vi "LEDShow.vi"(1 "DigntNumber":u32, 2 "InputNumber":dbl) -> (0 "MyLED":u16[](array[ring]))   [LabVIEW 2011]
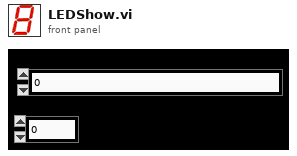
[diagram p1: front panel]
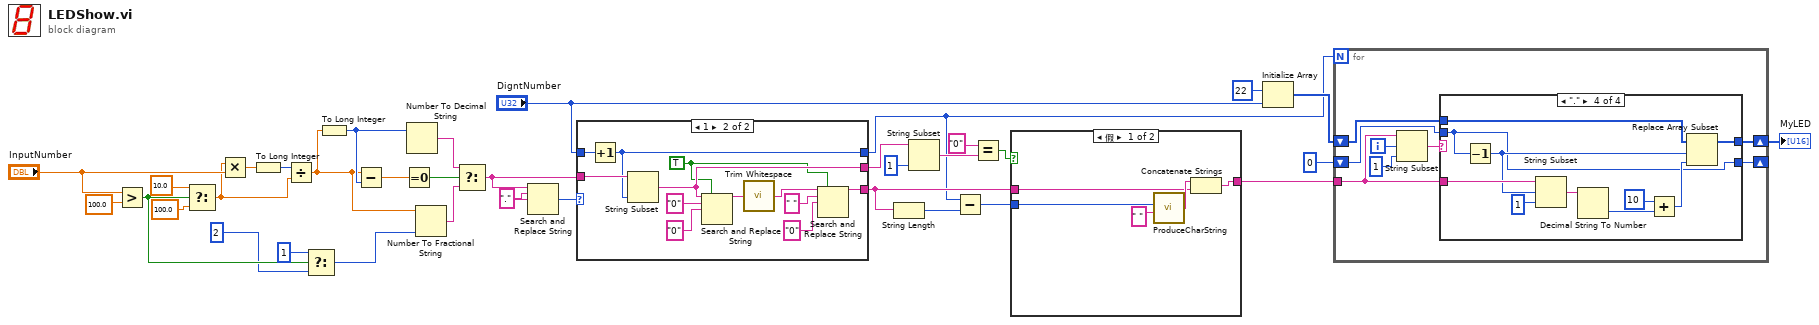
[diagram p0: block diagram]
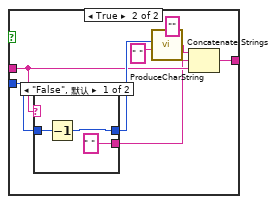
[diagram p3: hidden frame]
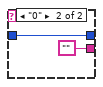
[diagram p4: hidden frame]
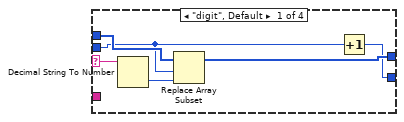
[diagram p5: hidden frame]
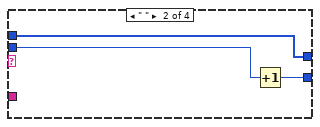
[diagram p6: hidden frame]
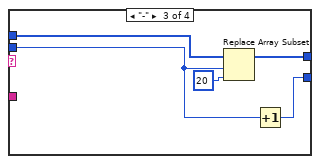
[diagram p7: hidden frame]
diagram:
  w35 = "." ("search string")
  n1 = Greater?(x="InputNumber", y=100.0 ("x")) -> (0:w4:bool)
  n2 = Select(t=10.0, s=w4, f=100.0 ("x")) -> (s? t:f=w5:dbl)
  n3 = Multiply(x=w5, y="InputNumber") -> (x*y=w12:dbl)
  n4 = To Long Integer(number=w12) -> (32bit integer=w10:i32)
  n5 = Divide(x=w10, y=w5) -> (x/y=w11:dbl)
  n6 = Select(t=i16 1, s=w4, f=i16 2 ("精度(6)")) -> (s? t:f=w2:i16)
  n7 = To Long Integer(number=w11) -> (32bit integer=w32:i32)
  n8 = Subtract(x=w11, y=w32) -> (x-y=w34:dbl)
  n9 = Equal To 0?(x=w34) -> (x = 0?=w33:bool)
  n10 = Number To Decimal String(number=w32) -> (decimal integer string=w31:string)  [unwired: 1 in]
  n11 = Number To Fractional String(number=w11, precision (6)=w2) -> (F-format string=w30:string)  [unwired: 2 in]
  n12 = Select(t=w31, s=w33, f=w30) -> (s? t:f=w29:string)
  n13 = Search and Replace String(input string=w29, search string=w35, replace string=w35) -> (number of replacements=w14:i32)  [unwired: 5 in, 3 out]
  n14 = case shown="1" w14 {
    tunnel: w29 -> [w36 w49]
    tunnel: [w36 w42] -> w26
    tunnel: "DigntNumber" -> [w37 w41]
    tunnel: [w36 w40] -> w20
    tunnel: [w37 w39] -> w15
    frame 0, Default {
    }
    frame 1 {
      w38 = TRUE ("replace all? (F)")
      n15 = Increment(x=w41) -> (x+1=w39:u32)
      n16 = String Subset(string=w49, length (rest)=w39) -> (substring=w40:string)  [unwired: 1 in]
      n17 = Search and Replace String(replace all?=w38, input string=w40, search string="0", replace string="0" ("replace string (\"\")")) -> (result string=w46:string)  [unwired: 4 in, 3 out]
      n18 = call <vilib>:"Trim Whitespace.vi"("string"=w46) -> ("trimmed string"=w45:string)  [unwired: 1 in]
      n19 = Search and Replace String(replace all?=w38, input string=w45, search string=" ", replace string="0" ("replace string (\"\")")) -> (result string=w42:string)  [unwired: 4 in, 3 out]
    }
  }
  n20 = String Length(string=w26) -> (length=w28:i32)
  n21 = String Subset(string=w20, length (rest)=1 ("length (rest)")) -> (substring=w19:string)  [unwired: 1 in]
  n22 = Subtract(x=w15, y=w28) -> (x-y=w27:u32)
  n23 = Equal?(x="0", y=w19) -> (x = y?=w17:bool)
  n24 = case shown="假" w17 {
    tunnel: w27 -> [w51 w59]
    tunnel: w26 -> [w52 w57]
    tunnel: [w50 w56] -> w13
    frame False {
      n25 = call "ProduceCharString.vi"("CharToBeProduce"=" ", "NumOfStr"=w51) -> ("ResultStr"=w53:string)  [unwired: 2 in]
      n26 = Concatenate Strings(w53, w52) -> (w50:string)
    }
    frame True {
      (unwired) "" ("字符串")
      n27 = case shown="\"False\", 默认" w57 {
        tunnel: w59 -> [w63 w66]
        tunnel: [w62 w66] -> w58
        tunnel: [" " ""] -> w55
        frame "False", Default {
          n28 = Decrement(x=w63) -> (x-1=w62:u32)
        }
        frame "0" {
        }
      }
      n29 = call "ProduceCharString.vi"("CharToBeProduce"=" ", "NumOfStr"=w58) -> ("ResultStr"=w60:string)  [unwired: 2 in]
      n30 = Concatenate Strings(w60, w55, w57) -> (w56:string)
    }
  }
  n31 = Initialize Array(u8 22, "DigntNumber") -> (w24:u8[])
  n32 = for {
    N: w15 -> [_]
    shift-right: [w73] -> w22
    shift-left: w24 -> [w74]
    tunnel: w13 -> [w70]
    shift-right: [w68] -> _
    shift-left: 0 -> [w69]
    i -> [w71]
    n33 = String Subset(string=w70, offset (0)=w71, length (rest)=1 ("length (rest)")) -> (substring=w67:string)
    n34 = case shown="\".\"" w67 {
      selector: w67 -> [w78 _ _ _]
      tunnel: w74 -> [w80 w83 w88 w97]
      tunnel: [w79 w83 w84 w98] -> w73
      tunnel: w69 -> [w75 w82 w86 w89]
      tunnel: w70 -> [_ _ _ w96]
      tunnel: [w76 w81 w87 w89] -> w68
      frame "digit", Default {
        n35 = Decimal String To Number(string=w78) -> (number=w77:i32)  [unwired: 2 in, 1 out]
        n36 = Replace Array Subset(array=w80, new element=w77, index=w75) -> (w79:u8[])
        n37 = Increment(x=w75) -> (x+1=w76:i32)
      }
      frame " " {
        n38 = Increment(x=w82) -> (x+1=w81:i32)
      }
      frame "-" {
        n39 = Replace Array Subset(array=w88, new element=u8 20 ("new element/subarray"), index=w86) -> (w84:u8[])
        n40 = Increment(x=w86) -> (x+1=w87:i32)
      }
      frame "." {
        n41 = Decrement(x=w89) -> (x-1=w90:i32)
        n42 = String Subset(string=w96, offset (0)=w90, length (rest)=1 ("length (rest)")) -> (substring=w94:string)
        n43 = Decimal String To Number(string=w94) -> (number=w93:i32)  [unwired: 2 in, 1 out]
        n44 = Add(x=10, y=w93) -> (x+y=w92:i32)
        n45 = Replace Array Subset(array=w97, new element=w92, index=w90) -> (w98:u8[])
      }
    }
  }
  "MyLED" <- w22
